vi "01_EMBALLAGE_BDD.vi"() -> ()   [LabVIEW 2020]
uses:
  EMBALLAGE_BDD_ongletPrincipal.ctl
  controles/enum_etatsMarche.ctl
  Modules/Fonction Standard/Bouton & Control/setget.ctl
  Modules/FS/60_FS_Controles/60_FS_SetGet.ctl
  Labview emballage/enum_ON_OFF_Lecteur.ctl
  <vilib>/Platform/browser.llb/Open URL in Default Browser (path).vi
  <vilib>/Utility/NIReport.llb/NI_ReportGenerationCore.lvlib
panel:
  out "PortCOM lecteur":refnum<visa-resource-name>
  out "Liste IP":string[](array[string])
  out "tableau":string[](array[string])
  in  "Pièces 2":string
  out "Error out":errorcluster
  out "Actualiser_lectureTableLocal":bool
  in  "ongletsPages":T1
  in  "Aide":bool caption="Help"
  in  "Error":errorcluster caption="Error in (no error)"
  out "Console":string
  out "Nom_PC":string
  out "Etat":string
  out "Sécurité OK":bool
  in  "initOK?":bool
  out "Version":string="En developpement"
  in  "btn_saferVersQuitter":bool
  in  "btn_safeVersMaintenance":bool
  in  "btn_safeVersInitialisation":bool
  in  "btn_maintenance_quitter":bool caption="Quitter Maintenance"
  in  "Cmd_onglets_maintenance":enum32{"Valeurs table bdd", "Initialisation"}(tab)
  out "Dec. Droite":string="^LH70,20"
  out "IP Imprimante Zebra":string(combo)
  out "PortCOM du lecteur":refnum<visa-resource-name> caption="PortCOM lecteur"
  in  "btn_Lecture_TableLocal":bool
  out "Imprimante certif":string(combo)
  out "Imprimante Zebra":string(combo)
  in  "Bouton Imprimer":bool
  in  "Imprimante Certificats":string(combo)
  in  "Param_Dec_Droit":bool
  in  "Dec.Droite":string="^LH70,20"
  in  "Init_Table_Hardware":bool
  in  "Imprimante Etiquettes":string(combo)
  in  "btn_choix_imprimante":bool
  in  "Btn_RechercherPortComScanner":bool
  out "Transfert_complete":bool
  out "Transfert":bool
  # "Valeurs des différentes éléments de la table SQlite local:"
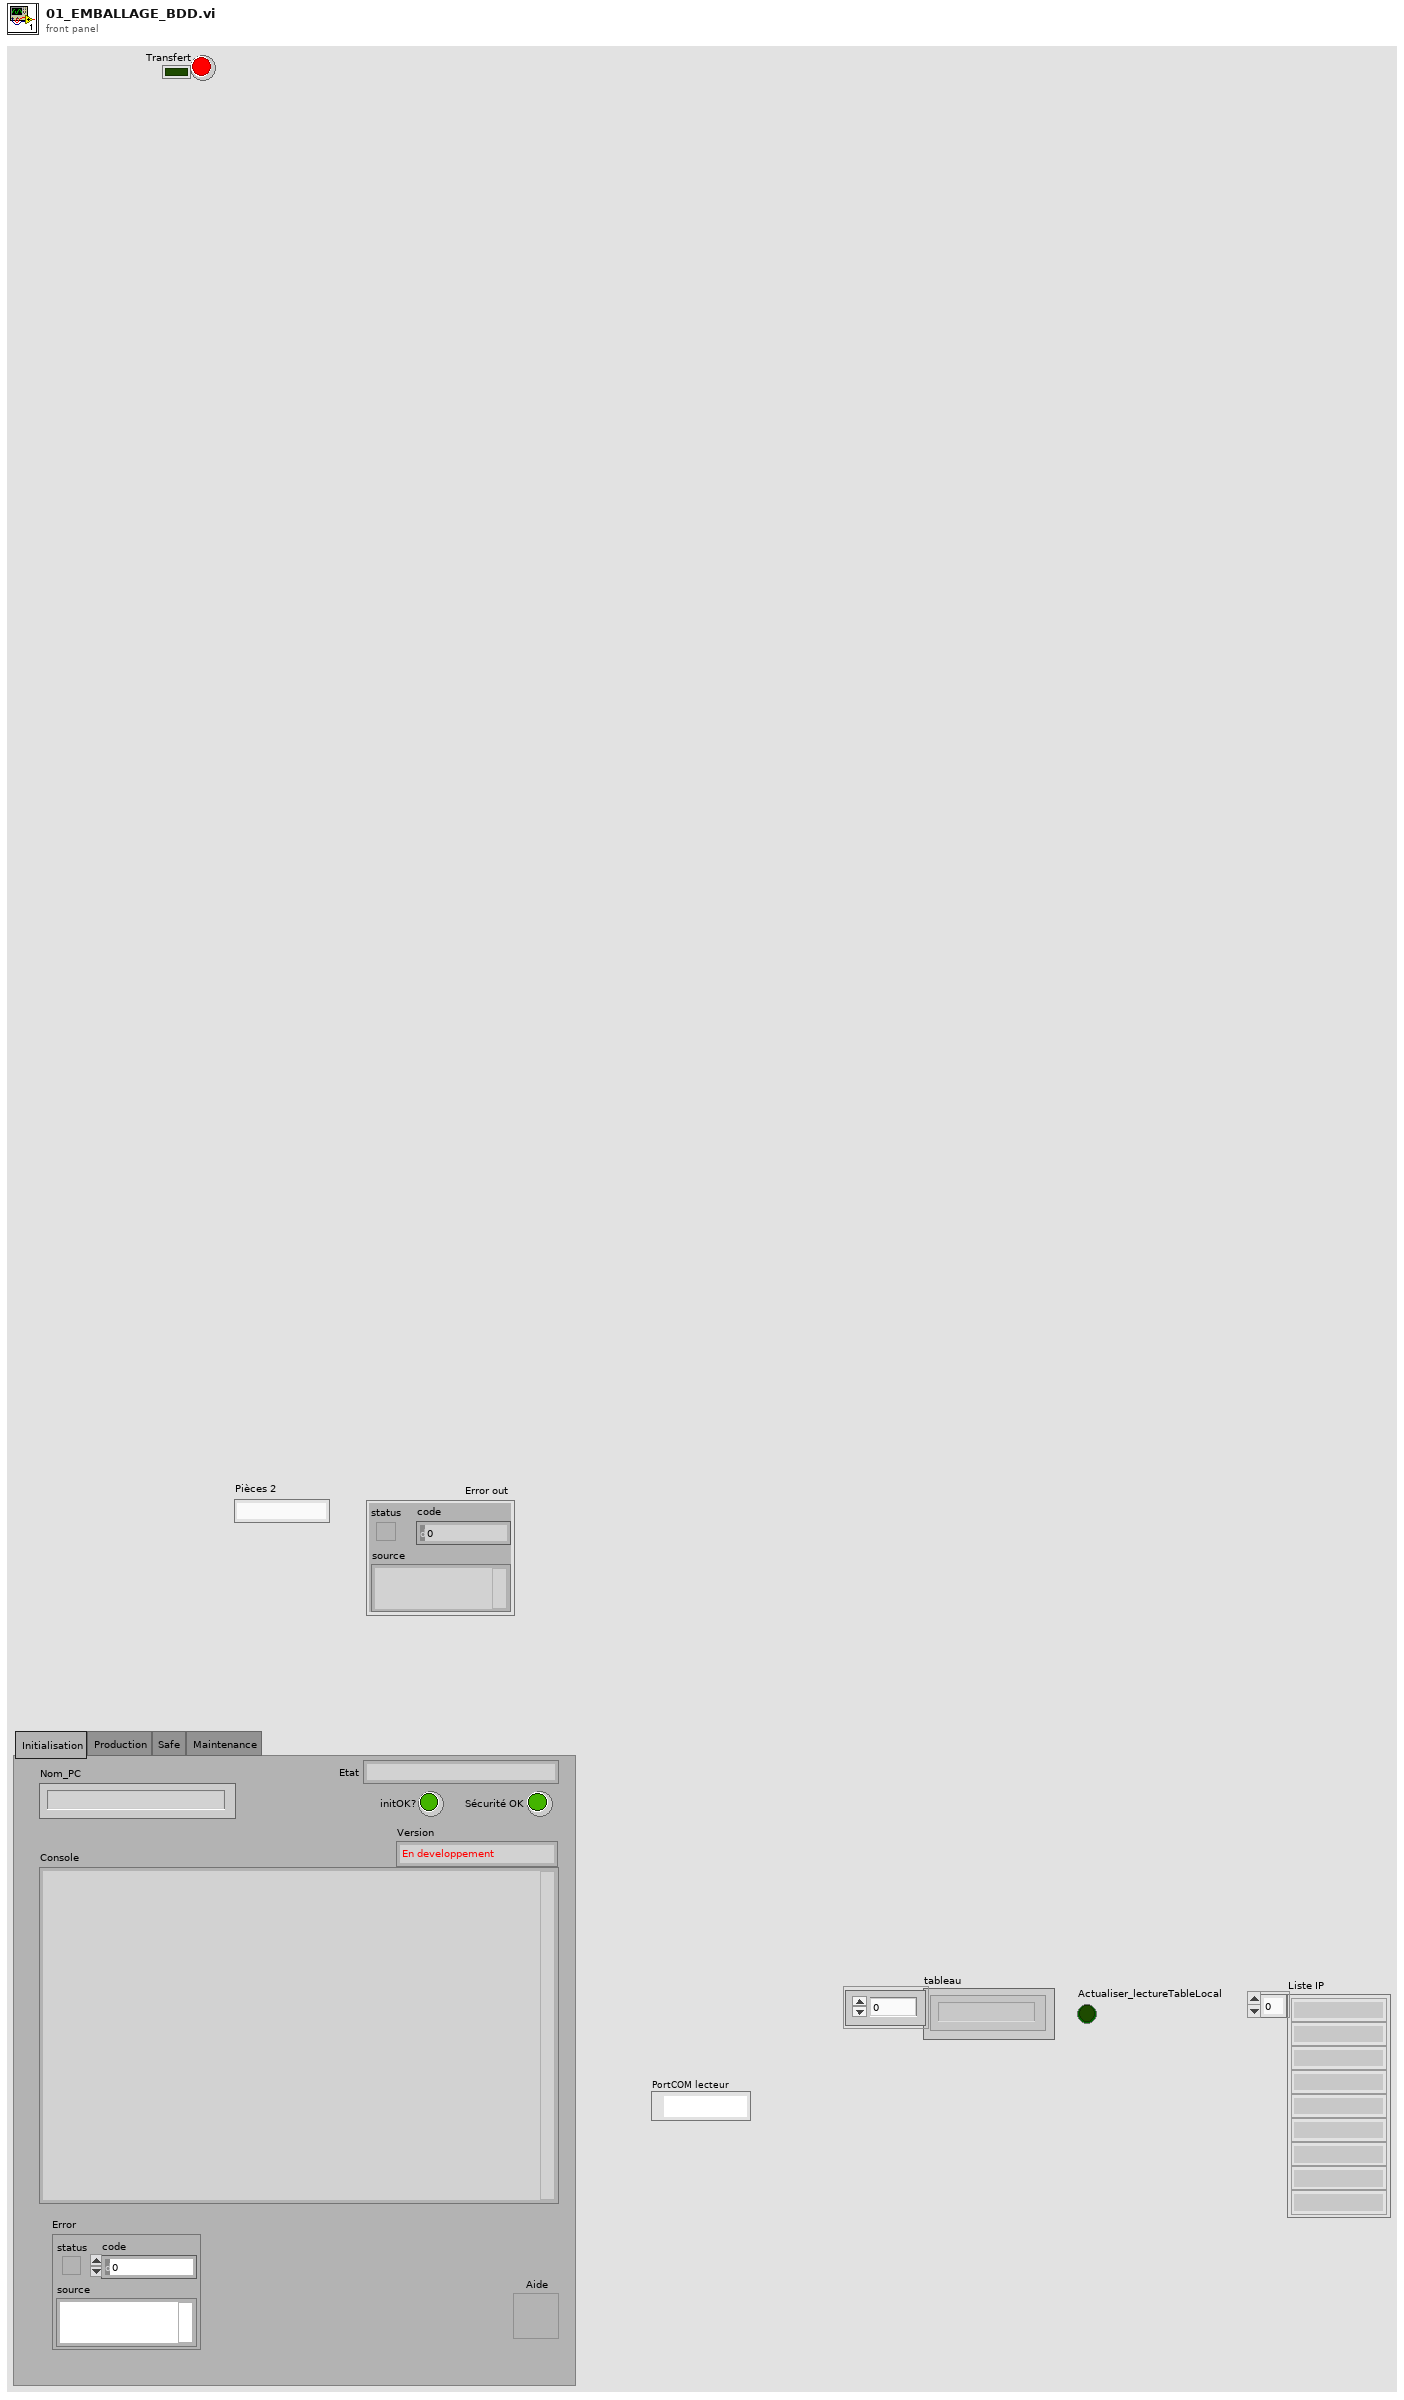
[diagram p1: front panel]
types:
  T1 = typedef "EMBALLAGE_BDD_ongletPrincipal.ctl" = enum32{"Initialisation", "Production", "Safe", "Maintenance"}
  T2 = typedef "enum_etatsMarche.ctl" = enum16{"initialisation", "safe", "armement", "production", "maintenance", "quitter"}
  T3 = typedef "60_FS_SetGet.ctl" = enum16{"set", "get"}
  T4 = typedef "setget.ctl" = enum16{"set", "get"}
  T5 = enum32{"Invalid", "Standard", "Closed", "Hidden", "Minimized", "Maximized"}
  T6 = typedef "enum_ON_OFF_Lecteur.ctl" = enum16{"ON_COURT", "OFF", "ON", "OFF (open/Close)", "ON (open/close)"}
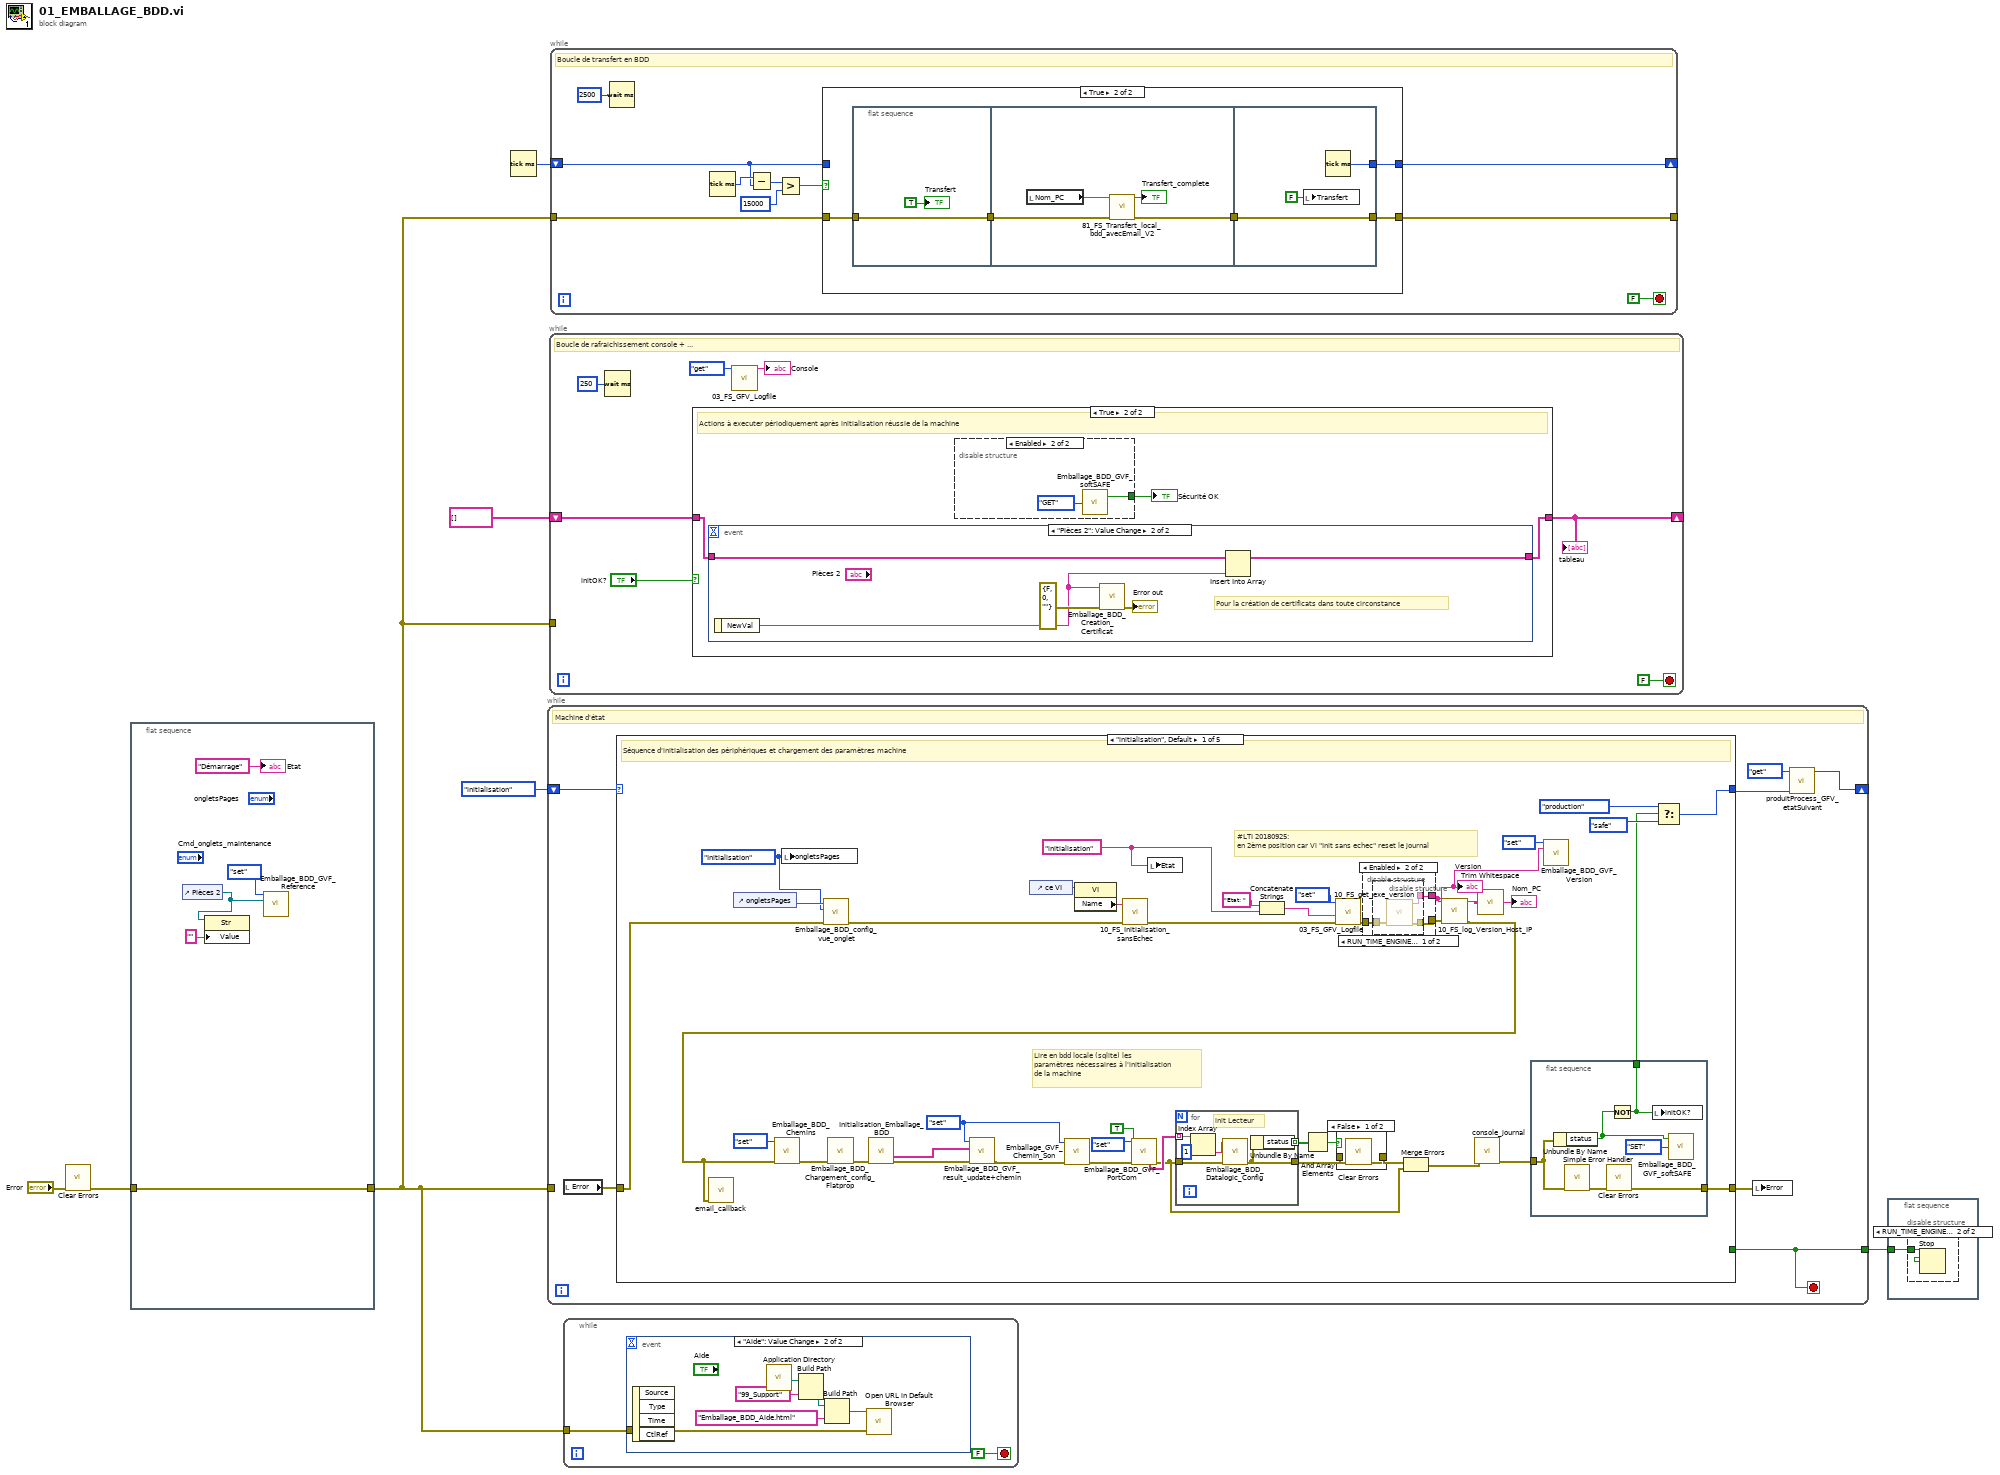
[diagram p0: block diagram]
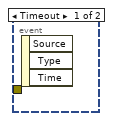
[diagram p2: hidden frame]
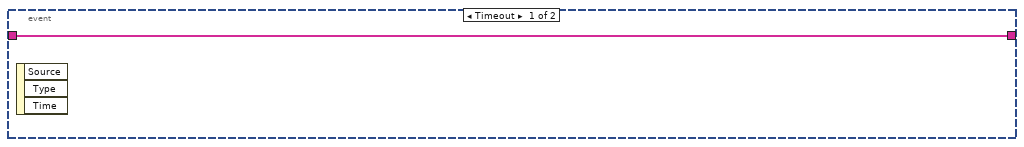
[diagram p5: hidden frame]
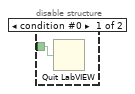
[diagram p7: hidden frame]
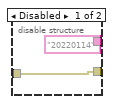
[diagram p8: hidden frame]
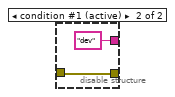
[diagram p9: hidden frame]
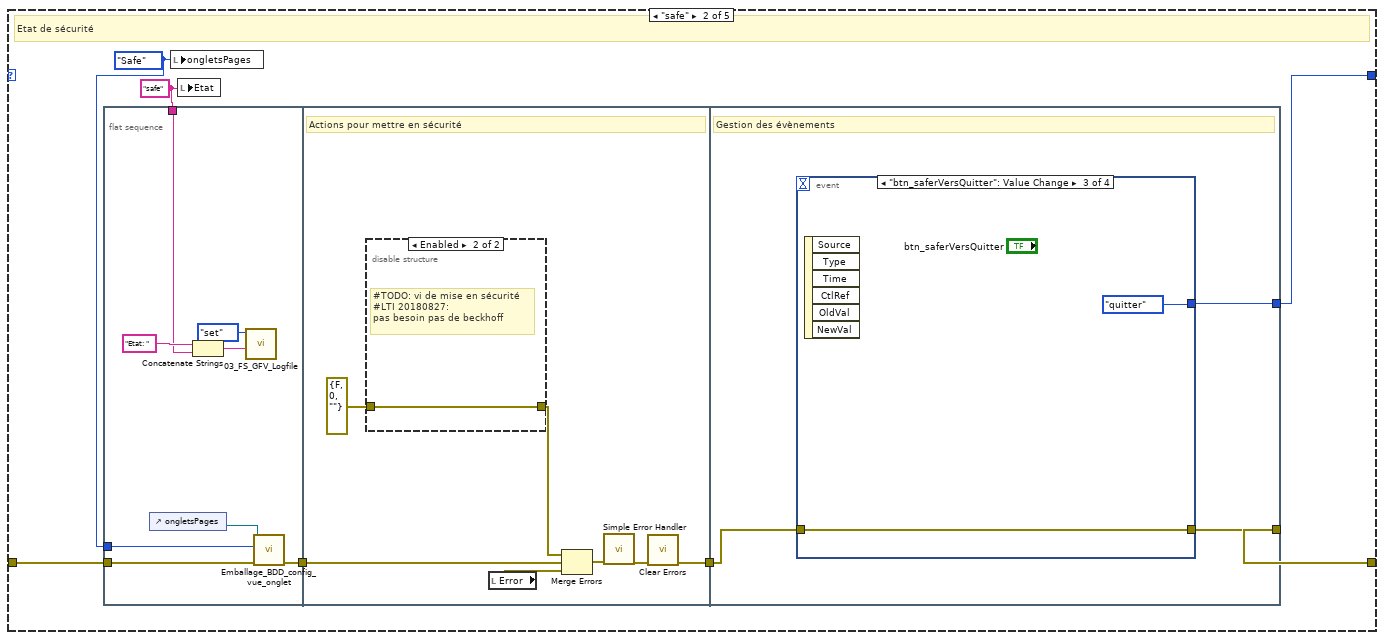
[diagram p11: hidden frame]
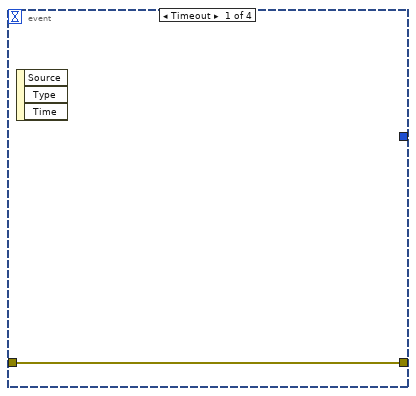
[diagram p13: hidden frame]
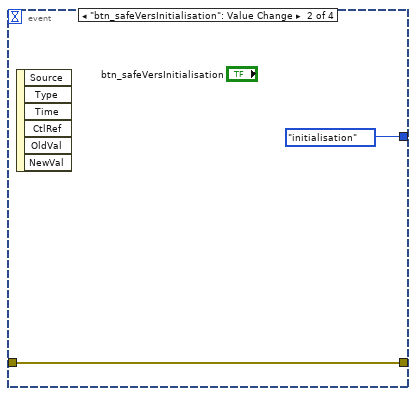
[diagram p14: hidden frame]
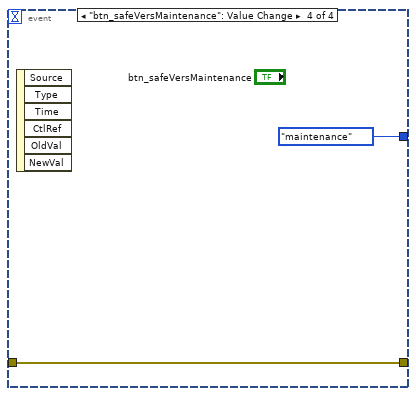
[diagram p15: hidden frame]
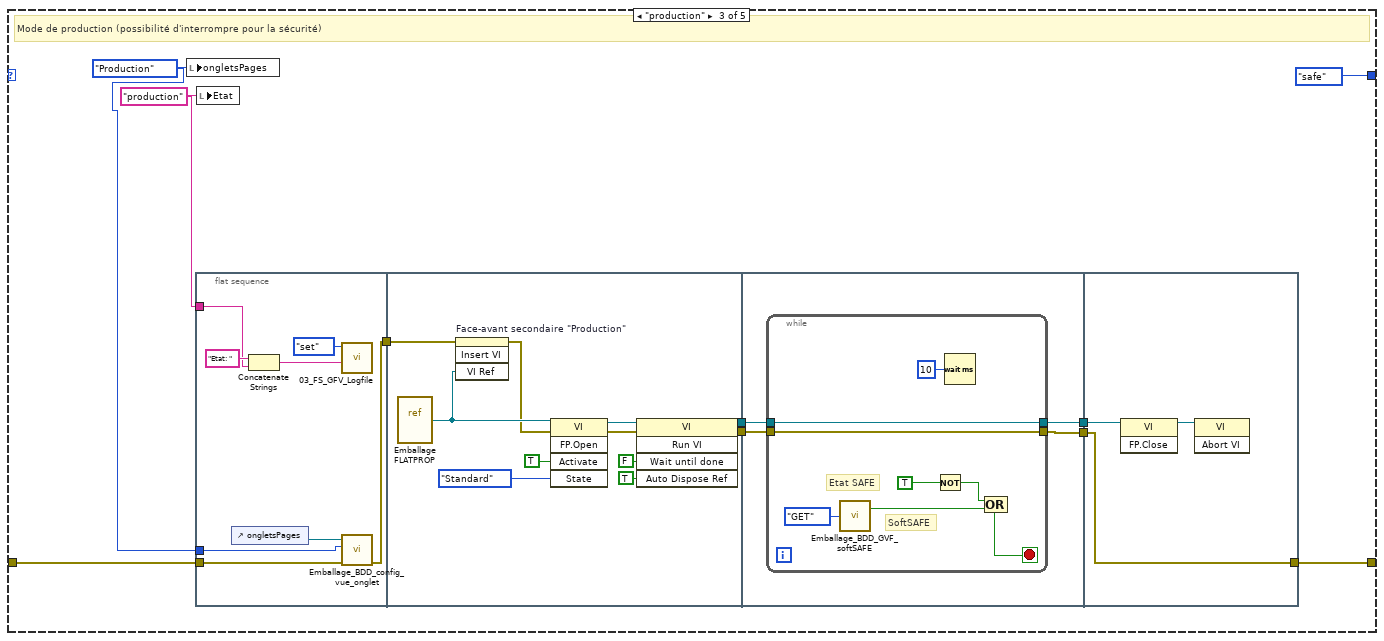
[diagram p16: hidden frame]
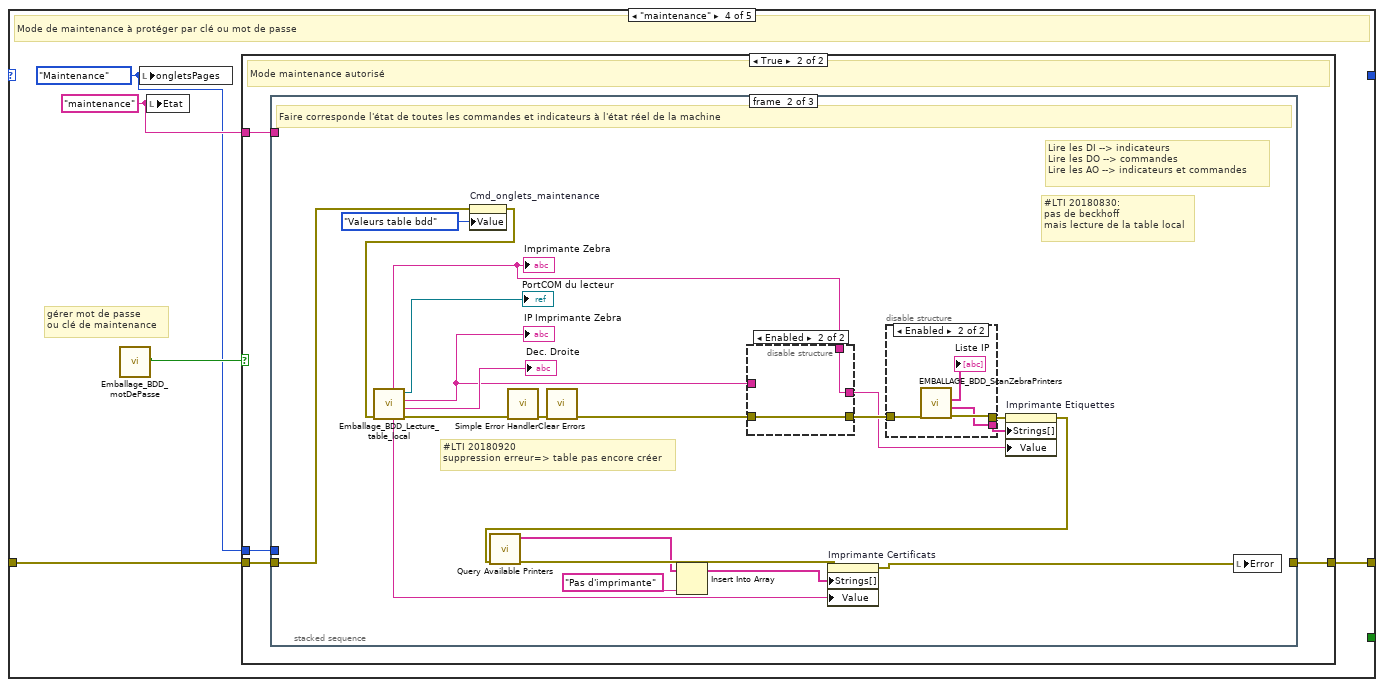
[diagram p17: hidden frame]
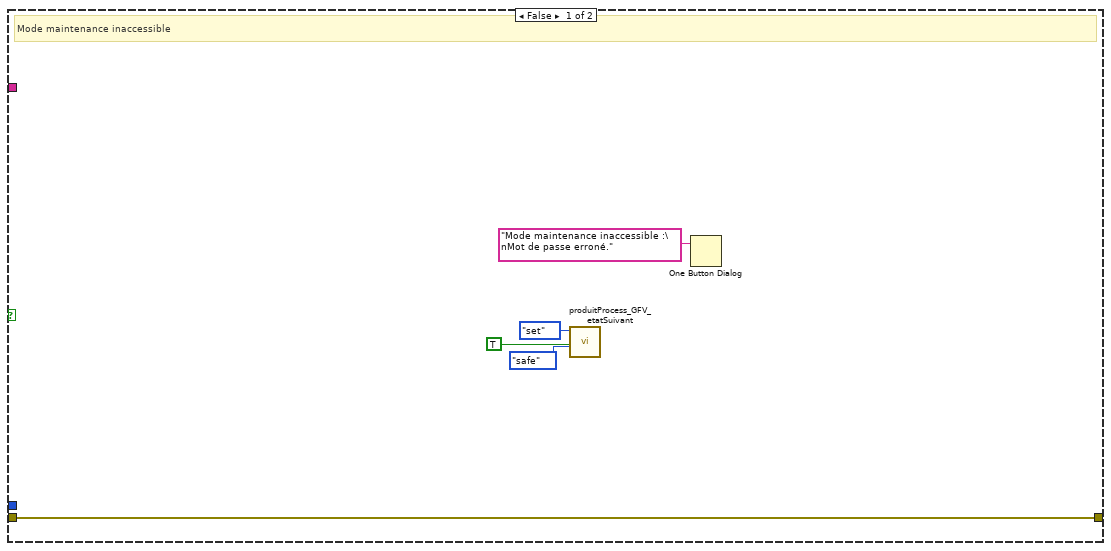
[diagram p18: hidden frame]
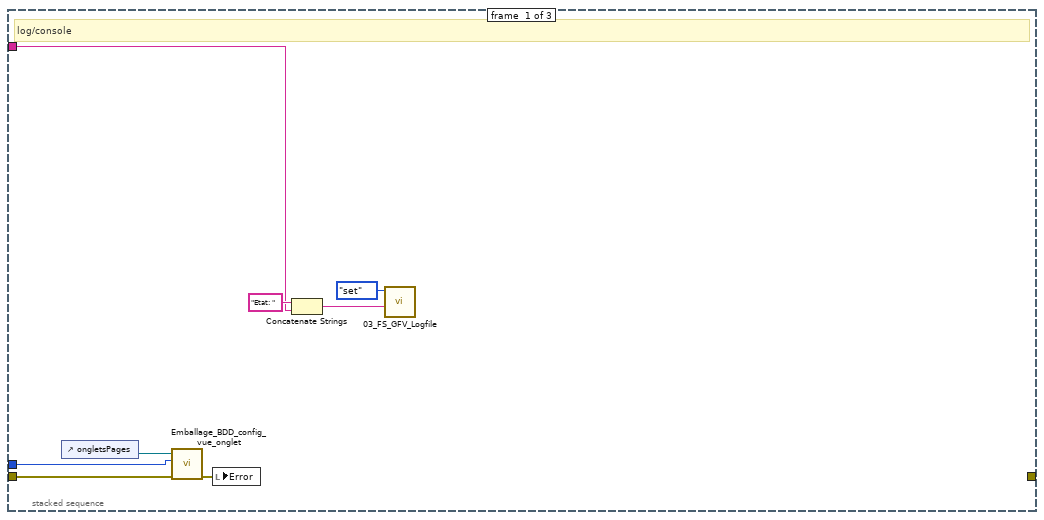
[diagram p19: hidden frame]
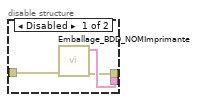
[diagram p20: hidden frame]
diagram:
  n1 = call <vilib>:"Clear Errors.vi"("error in (no error)"="Error") -> ("error out"=w4:errorcluster)  [unwired: 5 in, 1 out]
  n2 = flat-sequence {
    tunnel: [w12] -> w2
    tunnel: w4 -> [w12]
    frame #0 {
      n3 = control-ref of="Pièces 2"() -> (w9:refnum<vi>)
      n4 = property class="Str"(reference=w9, "Value"="" ("Valeur")) -> ()  [unwired: 1 in, 2 out]
      n5 = call "Emballage_BDD_GVF_Reference.vi"("SetGet"=60_FS_SetGet."set", "ref Piece IN"=w9) -> ()  [unwired: 12 in, 2 out]
      "Etat" <- "Démarrage" ("Etat")
    }
  }
  n6 = Tick Count (ms)() -> (millisecond timer value=w3:u32)
  n7 = while {
    tunnel: w2 -> [_]
    tunnel: [w18] -> w5
    shift-right: [w15] -> _
    shift-left: enum_etatsMarche."initialisation" -> [w19]
    stop <- w18 stop-if-true
    # "Machine d'état"
    n8 = local read "Error"() -> (w17:errorcluster)
    n9 = case shown="\"initialisation\", Default" w19 {
      tunnel: [_ _ _ _ TRUE] -> w18
      tunnel: [w58 w92 enum_etatsMarche."safe" _ _] -> w13
      tunnel: w17 -> [w37 w91 w127 w167 w325]
      tunnel: [w55 w89 w124 w168 w314] -> w16
      frame "initialisation", Default {
        w50 = enum16{"get", "set"}."set" ("Énum")
        w40 = "initialisation" ("Etat")
        w35 = EMBALLAGE_BDD_ongletPrincipal."Initialisation" ("ongletsPages")
        # "#LTI 20180925:\nen 2ème position car Vi \"Init sans echec\" reset le journal"
        # "Lire en bdd locale (sqlite) les\nparamètres nécessaires à l'initialisation\nde la machine"
        # "Séquence d'initialisation des périphériques et chargement des paramètres machine"
        n10 = control-ref of="ongletsPages"() -> (w38:refnum<vi>)
        n11 = local write "ongletsPages"(w35) -> ()
        n12 = call "Emballage_BDD_config_vue_onglet.vi"("entrée d'erreur (pas d'erreur)"=w37, "onglet_Actif"=w35, "TabControl en entrée"=w38) -> ("sortie d'erreur"=w36:errorcluster)  [unwired: 8 in]
        n13 = control-ref of="ce VI"() -> (w60:refnum<vi>)
        n14 = property class="VI"(reference=w60) -> ("Name"=w59:string)  [unwired: 1 in, 2 out]
        n15 = call "10_FS_Initialisation_sansEchec.vi"("error in (no error)"=w36, "01_Nom_Application.vi"=w59) -> ("error out"=w39:errorcluster)  [unwired: 8 in, 1 out]
        n16 = local write "Etat"(w40) -> ()
        n17 = Concatenate Strings("Etat: " ("chaîne"), w40) -> (w42:string)
        n18 = call "03_FS_GFV_Logfile.vi"("error in"=w39, "Chaîne"=w42, "States"=60_FS_SetGet."set") -> ("error out"=w21:errorcluster)  [unwired: 7 in, 1 out]
        n19 = disable-structure shown="Enabled" {
          disable-tunnel: ["20220114" ("Version") w63] -> w31
          disable-tunnel: [w61 w64] -> w22
          disable-tunnel: w21 -> [w61 w65]
          frame Disabled {
          }
          frame Enabled {
            n20 = disable-structure shown="RUN_TIME_ENGINE==True, Default" {
              disable-tunnel: w65 -> [w68 w70]
              disable-tunnel: [w67 w70] -> w64
              disable-tunnel: [w66 "dev" ("version")] -> w63
              frame condition #0 {
                n21 = call "10_FS_get_exe_version.vi"("error in"=w68) -> ("error out"=w67:errorcluster, "version"=w66:string)  [unwired: 8 in, 1 out]
              }
              frame condition #1 (active) {
              }
            }
          }
        }
        "Version" <- w31
        n22 = call "10_FS_log_Version_Host_IP.vi"("error in (no error)"=w22, "Version"=w31) -> ("error out"=w20:errorcluster, "hostname"=w33:string)  [unwired: 7 in, 1 out]
        n23 = call "email_callback.vi"("entrée d'erreur"=w20) -> ()  [unwired: 10 in, 1 out]
        n24 = call "Emballage_BDD_Chemins.vi"("error in (no error)"=w20, "SetGet"=60_FS_SetGet."set") -> ("error out"=w30:errorcluster)  [unwired: 8 in, 1 out]
        n25 = call "Emballage_BDD_Chargement_config_Flatprop.vi"("Error in"=w30) -> ("Error out"=w46:errorcluster)  [unwired: 10 in]
        n26 = call "Initialisation_Emballage_BDD.vi"("entrée d'erreur (pas d'erreur)"=w46) -> ("Tab codif-code bar"=w51:string[][], "sortie d'erreur"=w53:errorcluster)  [unwired: 12 in, 1 out]
        n27 = call "Emballage_BDD_GVF_result_update+chemin.vi"("Error in"=w53, "Tab codif-code bar IN"=w51, "Énum"=w50) -> ("Error out"=w52:errorcluster)  [unwired: 7 in, 1 out]
        n28 = call "Emballage_GVF_Chemin_Son.vi"("entrée d'erreur (pas d'erreur)"=w52, "Énum"=w50) -> ("sortie d'erreur"=w48:errorcluster)  [unwired: 5 in, 4 out]
        n29 = call "Emballage_BDD_GVF_PortCom.vi"("Énum"=enum16{"get", "set"}."set", "bdd"=TRUE, "Error in"=w48) -> ("Result Set"=w29:string[][], "Error out"=w27:errorcluster)  [unwired: 6 in, 5 out]
        n30 = for {
          tunnel: w27 -> [w79]
          tunnel: w29 -> [w76] mode=indexing
          tunnel: [w78] -> w25
          tunnel: [w77] -> w24 mode=indexing
          # "init Lecteur"
          n31 = Index Array(array=w76, index=1 ("indice")) -> (element=w74:string)
          n32 = call "Emballage_BDD_Datalogic_Config.vi"("error in (no error)"=w79, "VISA resource name"=w74) -> ("error out"=w78:errorcluster)  [unwired: 9 in]
          n33 = Unbundle By Name(w78) -> ("status"=w77:bool)
        }
        n34 = And Array Elements(Boolean array=w24) -> (logical AND=w23:bool)
        n35 = case shown="False" w23 {
          tunnel: [w72 w73] -> w26
          tunnel: w25 -> [w71 w73]
          frame False {
            n36 = call <vilib>:"Clear Errors.vi"("error in (no error)"=w71) -> ("error out"=w72:errorcluster)  [unwired: 5 in, 1 out]
          }
          frame True {
          }
        }
        n37 = Merge Errors(w26, w27) -> (w28:errorcluster)
        n38 = call "console_journal.vi"("entrée d'erreur (pas d'erreur)"=w28) -> ("sortie d'erreur"=w56:errorcluster)  [unwired: 10 in]
        n39 = call <vilib>:"Trim Whitespace.vi"("string"=w33) -> ("trimmed string"=→"Nom_PC":string)  [unwired: 1 in]
        n40 = flat-sequence {
          tunnel: w56 -> [w82]
          tunnel: [w85] -> w49
          tunnel: [w83] -> w55
          frame #0 {
            n41 = Unbundle By Name(w82) -> ("status"=w81:bool)
            n42 = call <vilib>:"Simple Error Handler.vi"("error in (no error)"=w82) -> ("error out"=w84:errorcluster)  [unwired: 4 in, 4 out]
            n43 = call <vilib>:"Clear Errors.vi"("error in (no error)"=w84) -> ("error out"=w83:errorcluster)  [unwired: 5 in, 1 out]
            n44 = Not(x=w81) -> (.not. x?=w85:bool)
            n45 = local write "initOK?"(w85) -> ()
            n46 = call "Emballage_BDD_GVF_softSAFE.vi"("Énum"=enum16{"SET", "GET"}."SET", "SOFTSAFE"=w81) -> ()  [unwired: 1 in, 2 out]
          }
        }
        n47 = call "Emballage_BDD_GVF_Version.vi"("SetGet"=60_FS_SetGet."set", "Version IN"=w31) -> ()  [unwired: 12 in, 2 out]
        n48 = Select(t=enum_etatsMarche."production", s=w49, f=enum_etatsMarche."safe") -> (s? t:f=w58:T2)
      }
      frame "safe" {
        w87 = "safe" ("Etat")
        w86 = EMBALLAGE_BDD_ongletPrincipal."Safe" ("ongletsPages")
        # "Etat de sécurité"
        n49 = flat-sequence {
          tunnel: w91 -> [w95]
          tunnel: [w94] -> w88
          tunnel: w87 -> [w97]
          tunnel: w86 -> [w93]
          tunnel: [w101] -> w90
          tunnel: w88 -> [w107]
          tunnel: [w112] -> w92
          tunnel: [w111] -> w89
          tunnel: w90 -> [w110]
          frame #0 {
            n50 = control-ref of="ongletsPages"() -> (w96:refnum<vi>)
            n51 = Concatenate Strings("Etat: " ("chaîne"), w97) -> (w99:string)
            n52 = call "03_FS_GFV_Logfile.vi"("Chaîne"=w99, "States"=60_FS_SetGet."set") -> ()  [unwired: 8 in, 2 out]
            n53 = call "Emballage_BDD_config_vue_onglet.vi"("entrée d'erreur (pas d'erreur)"=w95, "onglet_Actif"=w93, "TabControl en entrée"=w96) -> ("sortie d'erreur"=w94:errorcluster)  [unwired: 8 in]
          }
          frame #1 {
            # "Actions pour mettre en sécurité"
            n54 = disable-structure shown="Enabled" {
              disable-tunnel: [w108 w109] -> w106
              disable-tunnel: errorcluster {"status"=FALSE, "code"=0, "source"=""} ("entrée d'erreur") -> [w108 w109]
              frame Disabled {
              }
              frame Enabled {
                # "#TODO: vi de mise en sécurité\n#LTI 20180827:\npas besoin pas de beckhoff"
              }
            }
            n55 = local read "Error"() -> (w104:errorcluster)
            n56 = Merge Errors(w106, w107, w104) -> (w103:errorcluster)
            n57 = call <vilib>:"Simple Error Handler.vi"("error in (no error)"=w103) -> ("error out"=w102:errorcluster)  [unwired: 4 in, 4 out]
            n58 = call <vilib>:"Clear Errors.vi"("error in (no error)"=w102) -> ("error out"=w101:errorcluster)  [unwired: 5 in, 1 out]
          }
          frame #2 {
            # "Gestion des évènements"
            n59 = event shown="[2] \"btn_saferVersQuitter\": Value Change" {
              selector: _ -> [_ _ _ _]
              dyn-events: _ -> [_ _ _ _]
              timeout: _ -> [_ _ _ _]
              tunnel: [_ enum_etatsMarche."initialisation" enum_etatsMarche."quitter" enum_etatsMarche."maintenance"] -> w112
              tunnel: [w113 w114 w116 w118] -> w111
              tunnel: w110 -> [w113 w114 w116 w118]
              event Timeout {
                n60 = event-data() -> ()  [unwired: 1 in, 3 out]
              }
              event "btn_safeVersInitialisation": Value Change {
                n61 = event-data() -> ()  [unwired: 1 in, 6 out]
              }
              event "btn_saferVersQuitter": Value Change {
                n62 = event-data() -> ()  [unwired: 1 in, 6 out]
              }
              event "btn_safeVersMaintenance": Value Change {
                n63 = event-data() -> ()  [unwired: 1 in, 6 out]
              }
            }
          }
        }
        n64 = local write "ongletsPages"(w86) -> ()
        n65 = local write "Etat"(w87) -> ()
      }
      frame "production" {
        w121 = "production" ("Etat")
        w120 = EMBALLAGE_BDD_ongletPrincipal."Production" ("ongletsPages")
        # "Mode de production (possibilité d'interrompre pour la sécurité)"
        n66 = local write "ongletsPages"(w120) -> ()
        n67 = flat-sequence {
          tunnel: w127 -> [w132]
          tunnel: [w131] -> w122
          tunnel: w121 -> [w134]
          tunnel: w120 -> [w130]
          tunnel: [w140] -> w129
          tunnel: [w138] -> w126
          tunnel: w122 -> [w139]
          tunnel: [w152] -> w128
          tunnel: w129 -> [w151]
          tunnel: w126 -> [w150]
          tunnel: [w149] -> w125
          tunnel: w128 -> [w162]
          tunnel: [w161] -> w124
          tunnel: w125 -> [w161]
          frame #0 {
            n68 = control-ref of="ongletsPages"() -> (w133:refnum<vi>)
            n69 = Concatenate Strings("Etat: " ("chaîne"), w134) -> (w136:string)
            n70 = call "03_FS_GFV_Logfile.vi"("Chaîne"=w136, "States"=60_FS_SetGet."set") -> ()  [unwired: 8 in, 2 out]
            n71 = call "Emballage_BDD_config_vue_onglet.vi"("entrée d'erreur (pas d'erreur)"=w132, "onglet_Actif"=w130, "TabControl en entrée"=w133) -> ("sortie d'erreur"=w131:errorcluster)  [unwired: 8 in]
          }
          frame #1 {
            n72 = vi-ref "Emballage FLATPROP.vi"() -> (w142:refnum<vi>)
            n73 = invoke on="Face-avant secondaire \"Production\"" class="FAsec" method="Insert VI"(error in=w139, "VI Ref"=w142) -> (error out=w141:errorcluster)  [unwired: 2 in, 3 out]
            n74 = invoke class="VI" method="FP.Open"(reference=w142, error in=w141, "Activate"=TRUE ("Activer ?"), "State"=T5."Standard" ("État")) -> (reference out=w146:refnum<vi>, error out=w145:errorcluster)  [unwired: 1 in, 3 out]
            n75 = invoke class="VI" method="Run VI"(reference=w146, error in=w145, "Wait until done"=FALSE ("Attendre la fin"), "Auto Dispose Ref"=TRUE ("Supprimer la référence automatiquement")) -> (reference out=w140:refnum<vi>, error out=w138:errorcluster)  [unwired: 1 in, 3 out]
          }
          frame #2 {
            n76 = while {
              tunnel: [w157] -> w152
              tunnel: w151 -> [w157]
              tunnel: w150 -> [w154]
              tunnel: [w154] -> w149
              stop <- w156 stop-if-true
              # "SoftSAFE"
              # "Etat SAFE"
              n77 = call "Emballage_BDD_GVF_softSAFE.vi"("Énum"=enum16{"SET", "GET"}."GET") -> ("SOFTSAFE"=w160:bool)  [unwired: 2 in, 1 out]
              n78 = Not(x=TRUE) -> (.not. x?=w159:bool)
              n79 = Wait (ms)(milliseconds to wait=u32 10 ("attente (ms)")) -> ()  [unwired: 1 out]
              n80 = Compound Arithmetic op=OR ("Opérateur arithmétique")(w159, w160) -> (w156:bool)
            }
          }
          frame #3 {
            n81 = invoke class="VI" method="FP.Close"(reference=w162) -> (reference out=w163:refnum<vi>)  [unwired: 2 in, 2 out]
            n82 = invoke class="VI" method="Abort VI"(reference=w163) -> ()  [unwired: 2 in, 3 out]
          }
        }
        n83 = local write "Etat"(w121) -> ()
      }
      frame "maintenance" {
        w165 = "maintenance" ("Etat")
        w164 = EMBALLAGE_BDD_ongletPrincipal."Maintenance" ("ongletsPages")
        # "gérer mot de passe\nou clé de maintenance"
        # "Mode de maintenance à protéger par clé ou mot de passe"
        n84 = call "Emballage_BDD_motDePasse.vi"() -> ("Booléen"=w166:bool)  [unwired: 11 in]
        n85 = local write "ongletsPages"(w164) -> ()
        n86 = local write "Etat"(w165) -> ()
        n87 = case shown="True" w166 {
          tunnel: [w173 w177] -> w168
          tunnel: w167 -> [w173 w176]
          tunnel: w165 -> [_ w175]
          tunnel: w164 -> [_ w174]
          frame False {
            # "Mode maintenance inaccessible"
            n88 = call "produitProcess_GFV_etatSuivant.vi"("etatPrioritaire"=enum_etatsMarche."safe", "prioritaire?"=TRUE, "fonction"=setget."set") -> ()  [unwired: 7 in, 2 out]
            n89 = One Button Dialog(message="Mode maintenance inaccessible :\nMot de passe erroné.") -> ()  [unwired: 1 in, 1 out]
          }
          frame True {
            # "Mode maintenance autorisé"
            n90 = stacked-sequence {
              tunnel: w176 -> [w180 w197 w221]
              tunnel: [_ _ w220] -> w177
              tunnel: w175 -> [w182 _ _]
              tunnel: w174 -> [w178 _ _]
              frame #0 {
                # "log/console"
                n91 = control-ref of="ongletsPages"() -> (w181:refnum<vi>)
                n92 = call "Emballage_BDD_config_vue_onglet.vi"("entrée d'erreur (pas d'erreur)"=w180, "onglet_Actif"=w178, "TabControl en entrée"=w181) -> ("sortie d'erreur"=w179:errorcluster)  [unwired: 8 in]
                n93 = local write "Error"(w179) -> ()
                n94 = Concatenate Strings("Etat: " ("chaîne"), w182) -> (w184:string)
                n95 = call "03_FS_GFV_Logfile.vi"("Chaîne"=w184, "States"=60_FS_SetGet."set") -> ()  [unwired: 8 in, 2 out]
              }
              frame #1 {
                # "#LTI 20180920\nsuppression erreur=> table pas encore créer"
                # "#LTI 20180830:\npas de beckhoff\nmais lecture de la table local"
                # "Lire les DI --> indicateurs\nLire les DO --> commandes\nLire les AO --> indicateurs et commandes"
                # "Faire corresponde l'état de toutes les commandes et indicateurs à l'état réel de la machine"
                n96 = property on="Cmd_onglets_maintenance" class="TabCtl (strict)"(error in=w197, "Value"=enum32{"Valeurs table bdd", "Initialisation"}."Valeurs table bdd" ("Cmd_onglets_maintenance")) -> (error out=w196:errorcluster)  [unwired: 1 in, 1 out]
                n97 = call "Emballage_BDD_Lecture_table_local.vi"("entrée d'erreur (pas d'erreur)"=w196) -> ("sortie d'erreur"=w202:errorcluster, "Dec.Droite 2"=→"Dec. Droite":string, "Com Imprimante"=w199:string, "Refnum VISA en sortie"=→"PortCOM du lecteur":refnum<visa-resource-name>, "Imprimante certif"=w189:string, "Imprimante Zebra"=w186:string)  [unwired: 4 in, 1 out]
                "IP Imprimante Zebra" <- w199
                "Imprimante Zebra" <- w186
                n98 = call <vilib>:"Simple Error Handler.vi"("error in (no error)"=w202) -> ("error out"=w195:errorcluster)  [unwired: 4 in, 4 out]
                n99 = call <vilib>:"Clear Errors.vi"("error in (no error)"=w195) -> ("error out"=w194:errorcluster)  [unwired: 5 in, 1 out]
                n100 = disable-structure shown="Enabled" {
                  disable-tunnel: [w217 w219] -> w201
                  disable-tunnel: [w216 w218] -> w200
                  disable-tunnel: w199 -> [w215 _]
                  disable-tunnel: w194 -> [w214 w219]
                  disable-tunnel: w186 -> [_ w218]
                  frame Disabled {
                    n101 = call "Emballage_BDD_adresseIPImprimante_NomImprimante.vi"("Error in"=w214, "ADRESSE_IP"=w215) -> ("Error out"=w217:errorcluster, "NOM"=w216:string)  [unwired: 8 in]
                  }
                  frame Enabled {
                  }
                }
                n102 = disable-structure shown="Enabled" {
                  disable-tunnel: [w209 w211] -> w204
                  disable-tunnel: [w208 w212] -> w203
                  disable-tunnel: w201 -> [w207 w213]
                  frame Disabled {
                    n103 = call "Emballage_BDD_NOMImprimante.vi"("Error in"=w207) -> ("Error out"=w208:errorcluster, "élément"=w209:string[])  [unwired: 9 in]
                  }
                  frame Enabled {
                    n104 = call "EMBALLAGE_BDD_ScanZebraPrinters.vi"("error in (no error)"=w213) -> ("error out"=w212:errorcluster, "Liste Nom"=w211:string[], "Liste IP"=→"Liste IP":string[])  [unwired: 7 in, 1 out]
                  }
                }
                n105 = property on="Imprimante Etiquettes" class="CmbBox"(error in=w203, "Strings[]"=w204, "Value"=w200) -> (error out=w193:errorcluster)  [unwired: 1 in, 1 out]
                n106 = call <vilib>:"Query Available Printers.vi"("error in (no error)"=w193) -> ("error out"=w192:errorcluster, "system configured printers"=w190:string[])  [unwired: 8 in, 1 out]
                n107 = Insert Into Array(array=w190, new element="Pas d'imprimante" ("nouvel élément/sous-tableau")) -> (w188:string[])  [unwired: 1 in]
                n108 = property on="Imprimante Certificats" class="CmbBox"(error in=w192, "Strings[]"=w188, "Value"=w189) -> (error out=w191:errorcluster)  [unwired: 1 in, 1 out]
                n109 = local write "Error"(w191) -> ()
              }
              frame #2 {
                n110 = while {
                  tunnel: w221 -> [_]
                  tunnel: [w224] -> w220
                  stop <- w223 stop-if-true
                  # "Signalement et effacement\ndes erreurs en mode\nmaintenance"
                  n111 = local read "Error"() -> (w227:errorcluster)
                  n112 = event shown="[7] \"btn_choix_imprimante\": Value Change" {
                    selector: _ -> [_ _ _ _ _ _ _ _]
                    dyn-events: _ -> [_ _ _ _ _ _ _ _]
                    timeout: -1 -> [_ _ _ _ _ _ _ _]
                    tunnel: w227 -> [w228 w229 w235 w253 w258 w284 w288 w296]
                    tunnel: [w228 w229 w234 w249 w257 w283 w286 w298] -> w226
                    tunnel: [_ TRUE _ _ _ _ _ _] -> w223
                    event Timeout {
                      n113 = event-data() -> ()  [unwired: 1 in, 3 out]
                    }
                    event "btn_maintenance_quitter": Value Change {
                      n114 = event-data() -> ()  [unwired: 1 in, 6 out]
                      n115 = call "produitProcess_GFV_etatSuivant.vi"("etatPrioritaire"=enum_etatsMarche."safe", "prioritaire?"=TRUE, "fonction"=setget."set") -> ()  [unwired: 7 in, 2 out]
                    }
                    event "Btn_RechercherPortComScanner": Value Change {
                      n116 = event-data() -> ()  [unwired: 1 in, 6 out]
                      n117 = disable-structure shown="Enabled" {
                        disable-tunnel: w235 -> [w239 w247]
                        disable-tunnel: [w236 w246] -> w234
                        frame Disabled {
                          n118 = call <vilib>:"Set Busy.vi"("error in (no error)"=w239) -> ("error out"=w238:errorcluster)  [unwired: 9 in, 1 out]
                          n119 = invoke on="PortCOM lecteur" class="NomVISA" method="Reinit To Default"(error in=w238) -> (error out=w242:errorcluster)  [unwired: 2 in, 2 out]
                          n120 = call "Emballage_BDD_Scann_Datalogic.vi"("error in (no error)"=w242) -> ("COM Array"=w244:refnum<visa-resource-name>, "error out"=w245:errorcluster)  [unwired: 14 in, 3 out]
                          "PortCOM lecteur" <- w244
                          n121 = call "Emballage_BDD_update_PortCom.vi"("Error in"=w245, "champsCom"="ComScan", "PortCom"=w244) -> ("Error out"=w241:errorcluster)  [unwired: 8 in]
                          n122 = property on="Actualiser_lectureTableLocal" class="Bool (strict)"(error in=w241, "Val(Sgnl)"=TRUE ("Valeur (Signalisation)")) -> (error out=w237:errorcluster)  [unwired: 1 in, 1 out]
                          n123 = call <vilib>:"Unset Busy.vi"("error in (no error)"=w237) -> ("error out"=w236:errorcluster)  [unwired: 10 in]
                        }
                        frame Enabled {
                          n124 = call "Emballage_BDD_scann_portcom.vi"("error in (no error)"=w247) -> ("Error out"=w246:errorcluster)  [unwired: 10 in]
                        }
                      }
                    }
                    event "Param_Dec_Droit": Value Change {
                      n125 = event-data() -> ()  [unwired: 1 in, 6 out]
                      n126 = call "Emballage_BDD_update_PortCom.vi"("Error in"=w253, "champsCom"="DecDroit", "PortCom"="Dec.Droite") -> ("Error out"=w250:errorcluster)  [unwired: 8 in]
                      n127 = property on="Actualiser_lectureTableLocal" class="Bool (strict)"(error in=w250, "Val(Sgnl)"=TRUE ("Valeur (Signalisation)")) -> (error out=w249:errorcluster)  [unwired: 1 in, 1 out]
                    }
                    event "Bouton Imprimer": Value Change {
                      n128 = event-data() -> ()  [unwired: 1 in, 6 out]
                      n129 = call "Emballage_BDD_GVF_PortCom.vi"("Énum"=enum16{"get", "set"}."set", "bdd"=TRUE) -> ("PortCom imprimante OUT"=w254:refnum<visa-resource-name>)  [unwired: 7 in, 6 out]
                      n130 = local read "Dec.Droite"() -> (w263:string)
                      n131 = property class="Instr"(reference=w254, error in=w258) -> (error out=w261:errorcluster, "Rsrc Name"=w262:string)  [unwired: 1 out]
                      n132 = Format Into String(format string="~SD25\n^XA\n^POI\n^ML900\n^PQ1\n^KL3\n^SC9600,8,N,1,,N\n^PRA\n^LL1428\n^MMC\n^LH100,20\n%s\r^A@B,1,1,ARI001^FT695,150^FD10.04.2020^FS\r\r^A@B,1,1,ARI003.FNT^FT0,1060^FDDestinataire^FS^A@B,1,1,ARI004.FNT^FT0,780^FDEMS Electro Medical System^FS\r^A@B,1,1,ARI003.FNT^FT40,1060^FDNo commande^FS\r^A@B,1,1,ARI003.FNT^FT40,780^FDCF-08-0253/2^FS\r^A@B,1,1,ARI003.FNT^FT80,1060^FDQuantité^FS\r^A@B,1,1,ARI003.FNT^FT80,780^FD50/100^FS\r^A@B,1,1,ARI003.FNT^FT120,1060^FDVotre réf.^FS\r^A@B,1,1,ARI003.FNT^FT120,780^FDEL-360/03^FS\r^A@B,1,1,ARI003.FNT^FT200,1060^FDNo. valve :^FS\r^A@B,1,1,ARI003^FT235,990^FD(P/N)^FS\r^A@B,1,1,ARI003.FNT^FT0,795^FD:^FS\r^A@B,1,1,ARI003.FNT^FT40,795^FD:^FS\r^A@B,1,1,ARI003.FNT^FT80,795^FD:^FS\r^A@B,1,1,ARI003.FNT^FT120,795^FD:^FS\r\r^FT596,40\n^BY2,2.0\n^BCI,70,N,N,N\n^FDEL-360 03 08010801 50^FS\r^A@I,1,1,ARI003^FT508,0^FDEL-360 03 08010801 50^FS\r\r^A@B,1,1,ARI001^FT200,870^FD08010001, 08010002, 08010003, 08010004, 08010005^FS\r^A@B,1,1,ARI001^FT230,870^FD08010006, 08010007, 08010008, 08010009, 08010010^FS\r^A@B,1,1,ARI001^FT260,870^FD08010011, 08010012, 08010013, 08010014, 08010015^FS\r^A@B,1,1,ARI001^FT290,870^FD08010016, 08010017, 08010018, 08010019, 08010020^FS\r^A@B,1,1,ARI001^FT320,870^FD08010021, 08010022, 08010023, 08010024, 08010025^FS\r^A@B,1,1,ARI001^FT350,870^FD08010026, 08010027, 08010028, 08010029, 08010030^FS\r^A@B,1,1,ARI001^FT380,870^FD08010031, 08010032, 08010033, 08010034, 08010035^FS\r^A@B,1,1,ARI001^FT410,870^FD08010036, 08010037, 08010038, 08010039, 08010040^FS\r^A@B,1,1,ARI001^FT440,870^FD08010041, 08010042, 08010043, 08010044, 08010045^FS\r^A@B,1,1,ARI001^FT470,870^FD08010046, 08010047, 08010048, 08010049, 08010050^FS\r\r^FT520,1060\n^GB0,910,3^FS\n\n^FT700,1060\n^BXB,6,200\n^FD12-216C-04521 EQIFIL 417mA 14.4ohm;03838/08-01.07.01;1/2^FS\r^A@B,1,1,ARI002^FT570,800^FDNo article FAS :^FS\r^A@B,1,1,ARI005^FT605,800^FD12-216C-04521 EQIFIL 417mA 14.4ohm^FS\r\r^A@B,1,1,ARI002^FT660,800^FDNo commande FAS :^FS\r^A@B,1,1,ARI005^FT660,490^FD03838/08-01.07.01^FS\r^A@B,1,1,ARI002^FT695,800^FDCarton : ^FS\r^A@B,1,1,ARI005^FT695,680^FD1/2^FS\r\r\r^XZ\r" ("chaîne de format"), w263) -> (resulting string=w259:string)  [unwired: 2 in, 1 out]
                      n133 = call <vilib>:"Clear Errors.vi"("error in (no error)"=w261) -> ("error out"=w260:errorcluster)  [unwired: 5 in, 1 out]
                      n134 = case shown="\"Faux\", Default" w262 {
                        tunnel: w259 -> [w274 _]
                        tunnel: [w269 w276] -> w257
                        tunnel: w260 -> [w267 w276]
                        tunnel: w254 -> [w265 _]
                        frame "Faux", Default {
                          n135 = VISA Open(error in (no error)=w267, VISA resource name=w265) -> (VISA resource name=w268:refnum<visa-resource-name>, error out=w266:errorcluster)  [unwired: 3 in]
                          n136 = VISA Write(VISA resource name=w268, write buffer=w274, error in (no error)=w266) -> (VISA resource name out=w270:refnum<visa-resource-name>, error out=w271:errorcluster)  [unwired: 1 out]
                          n137 = VISA Clear(VISA resource name=w270, error in (no error)=w271) -> (VISA resource name out=w272:refnum<visa-resource-name>, error out=w273:errorcluster)
                          n138 = VISA Close(VISA resource name=w272, error in (no error)=w273) -> (error out=w269:errorcluster)
                        }
                        frame "" {
                          # "Fonctionne OK avec \nChoix imprim.  \"Sans_imprimante\"\net Visa: \"none\""
                          n139 = One Button Dialog(message="Veuillez sélectionner une imprimante") -> ()  [unwired: 1 in, 1 out]
                        }
                      }
                    }
                    event "btn_Lecture_TableLocal", "Actualiser_lectureTableLocal": Value Change {
                      n140 = event-data() -> ()  [unwired: 1 in, 6 out]
                      n141 = call "Emballage_BDD_Lecture_table_local.vi"("entrée d'erreur (pas d'erreur)"=w284) -> ("sortie d'erreur"=w283:errorcluster, "Dec.Droite 2"=w282:string, "Com Imprimante"=w281:string, "Refnum VISA en sortie"=w280:refnum<visa-resource-name>, "Imprimante certif"=→"Imprimante certif":string, "Imprimante Zebra"=w277:string)  [unwired: 4 in, 1 out]
                      n142 = local write "IP Imprimante Zebra"(w281) -> ()
                      n143 = local write "Imprimante Zebra"(w277) -> ()
                      n144 = local write "PortCOM du lecteur"(w280) -> ()
                      n145 = local write "Dec. Droite"(w282) -> ()
                      "Actualiser_lectureTableLocal" <- FALSE ("LectuteTableLocal")
                    }
                    event "Init_Table_Hardware": Value Change {
                      n146 = event-data() -> ()  [unwired: 1 in, 6 out]
                      n147 = call "Emballage_BDD_bdd_initHardware.vi"("error in (no error)"=w288) -> ("error out"=w287:errorcluster)  [unwired: 10 in]
                      n148 = property on="Actualiser_lectureTableLocal" class="Bool (strict)"(error in=w287, "Val(Sgnl)"=TRUE ("Valeur (Signalisation)")) -> (error out=w286:errorcluster)  [unwired: 1 in, 1 out]
                    }
                    event "btn_choix_imprimante": Value Change {
                      n149 = event-data() -> ()  [unwired: 1 in, 6 out]
                      n150 = disable-structure shown="Enabled" {
                        disable-tunnel: [w307 w312] -> w304
                        disable-tunnel: [w306 w311] -> w303
                        disable-tunnel: w296 -> [w305 w312]
                        disable-tunnel: "Imprimante Etiquettes" -> [_ w309]
                        frame Disabled {
                          n151 = call "Imprimante sélection_bdd.vi"("entrée d'erreur"=w305) -> ("sortie d'erreur"=w307:errorcluster, "Output ressource VISA"=w306:refnum<visa-resource-name>)  [unwired: 1 in]
                        }
                        frame Enabled {
                          n152 = property on="Imprimante Etiquettes" class="CmbBox"() -> ("Strings[]"=w310:string[])  [unwired: 2 in, 2 out]
                          n153 = local read "Liste IP"() -> (w313:string[])
                          n154 = Search 1D Array(1D array=w310, element=w309) -> (index of element=w308:i32)  [unwired: 1 in]
                          n155 = call "EMBALLAGE_BDD_ZebraPrinter_IPComplet.vi"("Liste IP"=w313, "indice"=w308) -> ("IP Zebra complet"=w311:string)
                        }
                      }
                      n156 = call "Emballage_BDD_update_PortCom.vi"("Error in"=w304, "champsCom"="ComImprimante", "PortCom"=w303) -> ("Error out"=w292:errorcluster)  [unwired: 8 in]
                      n157 = call "Emballage_BDD_update_PortCom.vi"("Error in"=w292, "champsCom"="NomImprimante", "PortCom"="Imprimante Etiquettes") -> ("Error out"=w291:errorcluster)  [unwired: 8 in]
                      n158 = call "Emballage_BDD_update_PortCom.vi"("Error in"=w291, "champsCom"="ImprimanteCertif", "PortCom"="Imprimante Certificats") -> ("Error out"=w295:errorcluster)  [unwired: 8 in]
                      n159 = Format Into String(format string="Imprimante Etiquette par défaut:\n%s\nImprimante Cerif. par défaut:\n%s" ("Message"), "Imprimante Etiquettes", "Imprimante Certificats") -> (resulting string=w300:string)  [unwired: 2 in, 1 out]
                      n160 = call "Afficher un message à l'utilisateur"("error in (no error)"=w295, "Message"=w300) -> ("error out"=w299:errorcluster)  [unwired: 8 in, 1 out]
                      n161 = property on="Actualiser_lectureTableLocal" class="Bool (strict)"(error in=w299, "Val(Sgnl)"=TRUE ("Valeur (Signalisation)")) -> (error out=w298:errorcluster)  [unwired: 1 in, 1 out]
                    }
                  }
                  n162 = call <vilib>:"Simple Error Handler.vi"("error in (no error)"=w226) -> ("error out"=w225:errorcluster)  [unwired: 4 in, 4 out]
                  n163 = call <vilib>:"Clear Errors.vi"("error in (no error)"=w225) -> ("error out"=w224:errorcluster)  [unwired: 5 in, 1 out]
                  n164 = local write "Error"(w224) -> ()
                }
              }
            }
          }
        }
      }
      frame "quitter" {
        # "#TODO : gèrer les fermeture des ports com ouverts etc..."
        # "Basculer softSAFE à FAUX"
        # "Quitter et proposer d'éteindre le PC"
        n165 = call "03_FS_GFV_Logfile.vi"("error in"=w325, "Chaîne"="Quitter", "States"=60_FS_SetGet."set") -> ("error out"=w324:errorcluster)  [unwired: 7 in, 1 out]
        n166 = local read "Nom_PC"() -> (w329:string)
        n167 = call "81_FS_Transfert_local_bdd.vi"("error in (no error)"=w324, "No_machine"=w329) -> ("error out (no error)"=w322:errorcluster, "Transfert_complete"=w328:bool)  [unwired: 8 in]
        n168 = local write "Transfert_complete"(w328) -> ()
        n169 = call "Emballage_BDD_GVF_softSAFE.vi"("Error in"=w322, "Énum"=enum16{"SET", "GET"}."SET", "SOFTSAFE"=FALSE) -> ("Error out"=w320:errorcluster)  [unwired: 1 out]
        n170 = call "Emballage_BDD_ON_OFF_Lecteur.vi"("Error in"=w320, "ON/OFF lecteur"=enum_ON_OFF_Lecteur."OFF (open/Close)") -> ("Error out"=w316:errorcluster)  [unwired: 7 in, 2 out]
        n171 = call "Emballage_BDD_GVF_PortCom.vi"("Énum"=enum16{"get", "set"}."get", "Error in"=w316) -> ("PortCom imprimante OUT"=w318:refnum<visa-resource-name>, "Error out"=w317:errorcluster)  [unwired: 7 in, 5 out]
        n172 = VISA Close(VISA resource name=w318, error in (no error)=w317) -> (error out=w314:errorcluster)
        n173 = call "email_stopWorker.vi"("entrée d'erreur (pas d'erreur)"=w314) -> ()  [unwired: 10 in, 1 out]
      }
    }
    n174 = local write "Error"(w16) -> ()
    n175 = call "produitProcess_GFV_etatSuivant.vi"("etatNormal"=w13, "fonction"=setget."get") -> ("etatSuivant"=w15:T2)  [unwired: 8 in, 1 out]
  }
  n176 = while {
    tunnel: w2 -> [_]
    shift-right: [w331] -> _
    shift-left: string[] [] ("tableau") -> [w332]
    stop <- FALSE stop-if-true
    # "Boucle de rafraichissement console + ..."
    n177 = Wait (ms)(milliseconds to wait=u32 250 ("attente (ms)")) -> ()  [unwired: 1 out]
    n178 = case shown="True" "initOK?" {
      tunnel: w332 -> [w338 w340]
      tunnel: [w338 w339] -> w331
      frame False {
      }
      frame True {
        # "Actions à executer périodiquement après initialisation réussie de la machine"
        n179 = event shown="[1] \"Pièces 2\": Value Change" {
          selector: _ -> [_ _]
          dyn-events: _ -> [_ _]
          timeout: _ -> [_ _]
          tunnel: w340 -> [w342 w345]
          tunnel: [w342 w344] -> w339
          event Timeout {
            n180 = event-data() -> ()  [unwired: 1 in, 3 out]
          }
          event "Pièces 2": Value Change {
            # "Pour la création de certificats dans toute circonstance"
            n181 = event-data() -> ("NewVal"=w343:string)  [unwired: 1 in]
            n182 = call "Emballage_BDD_Creation_Certificat.vi"("Error in"=errorcluster {"status"=FALSE, "code"=0, "source"=""}, "CODE BARRE du produit correspondant au certificat"=w343) -> ("Error out"=→"Error out":errorcluster)  [unwired: 9 in]
            n183 = Insert Into Array(array=w345, new element=w343) -> (w344:string[])  [unwired: 1 in]
          }
        }
        n184 = disable-structure shown="Enabled" {
          disable-tunnel: [_ w348] -> w341
          frame Disabled {
            # "Rafraichissement de l'état de sécurité\n(Lecture DI)"
          }
          frame Enabled {
            n185 = call "Emballage_BDD_GVF_softSAFE.vi"("Énum"=enum16{"SET", "GET"}."GET") -> ("SOFTSAFE"=w348:bool)  [unwired: 2 in, 1 out]
          }
        }
        "Sécurité OK" <- w341
      }
    }
    "tableau" <- w331
    n186 = call "03_FS_GFV_Logfile.vi"("States"=60_FS_SetGet."get") -> ("Log file"=→"Console":string)  [unwired: 9 in, 1 out]
  }
  n187 = while {
    tunnel: w2 -> [w359]
    tunnel: [w358] -> _
    shift-right: [w356] -> _
    shift-left: w3 -> [w351]
    stop <- FALSE stop-if-true
    # "Boucle de transfert en BDD"
    n188 = Wait (ms)(milliseconds to wait=u32 2500 ("attente (ms)")) -> ()  [unwired: 1 out]
    n189 = Tick Count (ms)() -> (millisecond timer value=w355:u32)
    n190 = Subtract(x=w355, y=w351) -> (x-y=w354:u32)
    n191 = Greater?(x=w354, y=u32 15000) -> (0:w352:bool)
    n192 = case shown="True" w352 {
      tunnel: w359 -> [w360 w364]
      tunnel: [w360 w363] -> w358
      tunnel: [w361 w362] -> w356
      tunnel: w351 -> [w361 _]
      frame False {
      }
      frame True {
        n193 = flat-sequence {
          tunnel: w364 -> [w368]
          tunnel: [w368] -> w366
          tunnel: [w371] -> w365
          tunnel: w366 -> [w372]
          tunnel: w365 -> [w375]
          tunnel: [w375] -> w363
          tunnel: [w373] -> w362
          frame #0 {
            "Transfert" <- TRUE ("transfert")
          }
          frame #1 {
            n194 = local read "Nom_PC"() -> (w369:string)
            n195 = call "81_FS_Transfert_local_bdd_avecEmail_V2.vi"("error in (no error)"=w372, "No_machine"=w369) -> ("error out (no error)"=w371:errorcluster, "Transfert_complete"=→"Transfert_complete":bool)  [unwired: 8 in]
          }
          frame #2 {
            n196 = local write "Transfert"(FALSE ("transfert")) -> ()
            n197 = Tick Count (ms)() -> (millisecond timer value=w373:u32)
          }
        }
      }
    }
  }
  n198 = while {
    tunnel: w2 -> [w377]
    stop <- FALSE stop-if-true
    n199 = event shown="[1] \"Aide\": Value Change" {
      selector: _ -> [_ _]
      dyn-events: _ -> [_ _]
      timeout: _ -> [_ _]
      tunnel: w377 -> [_ w379]
      event Timeout {
        n200 = event-data() -> ()  [unwired: 1 in, 3 out]
      }
      event "Aide": Value Change {
        n201 = event-data() -> ()  [unwired: 1 in, 4 out]
        n202 = call <vilib>:"Application Directory.vi"() -> ("Application Directory"=w383:path)
        n203 = Build Path(base path=w383, name or relative path="99_Support" ("nom ou chemin relatif")) -> (appended path=w381:path)
        n204 = Build Path(base path=w381, name or relative path="Emballage_BDD_Aide.html" ("nom ou chemin relatif")) -> (appended path=w378:path)
        n205 = call-poly <vilib>:"Open URL in Default Browser.vi"("error in (no error)"=w379, "path"=w378) -> ()  [unwired: 4 in, 2 out]
      }
    }
  }
  n206 = flat-sequence {
    tunnel: w5 -> [w384]
    frame #0 {
      n207 = disable-structure shown="RUN_TIME_ENGINE==False" {
        disable-tunnel: w384 -> [w385 w386]
        frame condition #0 {
          n208 = Quit LabVIEW(quit? (T)=w385) -> ()
        }
        frame condition #1 (active) {
          n209 = Stop(stop? (T)=w386) -> ()
        }
      }
    }
  }
